vi "CropOutOfBound.vi"(11 "image data in":T1) -> (3 "image data out":T1)   [LabVIEW 2021, in "Picture2D.lvlib"]
uses:
  Picture2D/Picture2D.lvlib
  <vilib>/picture/picture.llb/imagedata.ctl
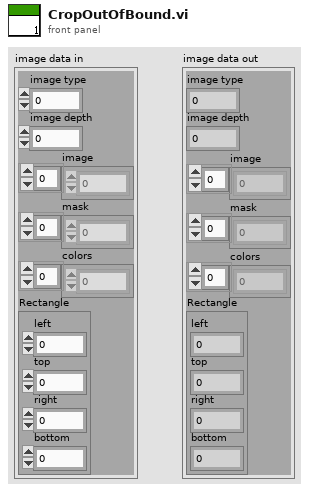
[diagram p1: front panel]
types:
  T1 = typedef "imagedata.ctl" = cluster{"image type":i32, "image depth":i32, "image":u8[], "mask":u8[], "colors":u32[], "Rectangle":cluster{"left":i16, "top":i16, "right":i16, "bottom":i16}}
  T2 = cluster{"left":i16, "top":i16, "right":i16, "bottom":i16}
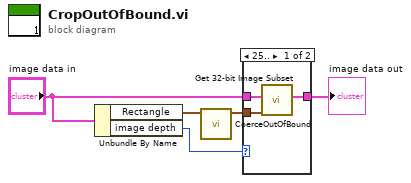
[diagram p0: block diagram]
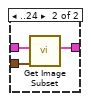
[diagram p2: hidden frame]
diagram:
  n1 = Unbundle By Name("image data in") -> ("Rectangle"=w2:T2, "image depth"=w1:i32)
  n2 = call "CoerceOutOfBound.vi"("Rectangle"=w2) -> ("Coerced Rectangle"=w3:T2)  [unwired: 10 in]
  n3 = case shown="25.." w1 {
    tunnel: w3 -> [w6 w9]
    tunnel: "image data in" -> [w8 w11]
    tunnel: [w7 w10] -> w5
    frame 25.. {
      n4 = call "Get 32-bit Image Subset.vi"("subset rect"=w6, "image data"=w8) -> ("image subset"=w7:T1)  [unwired: 4 in, 1 out]
    }
    frame ..24 {
      n5 = call <vilib>:"Get Image Subset.vi"("subset rect"=w9, "image data"=w11) -> ("image subset"=w10:T1)  [unwired: 4 in, 1 out]
    }
  }
  "image data out" <- w5
